vi "Mock Command.vi"(8 "error in (no error)":errorcluster, 11 "VISA Resource in":refnum<visa-resource-name>) -> (0 "error out":errorcluster, 1 "Fake Output":dbl, 3 "VISA Resource out":refnum<visa-resource-name>)   [LabVIEW 2020, in "plugin_flodx_pressure.lvlib" / "mock_driver.lvlib"]
doc: "Example of a mock or dummy driver VI which is meant to be called within plugin.lvlib in place of real instrument drivers as a development/debugging tool where hardware access may not be possible or convienent."
uses:
  mock_driver.lvlib
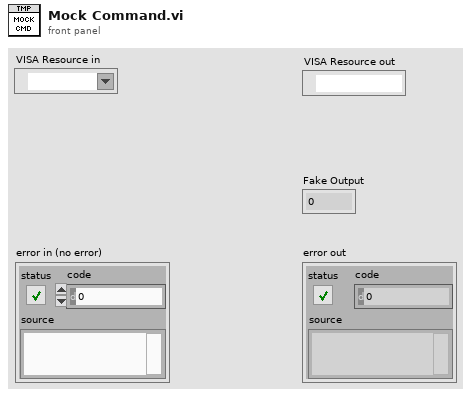
[diagram p1: front panel]
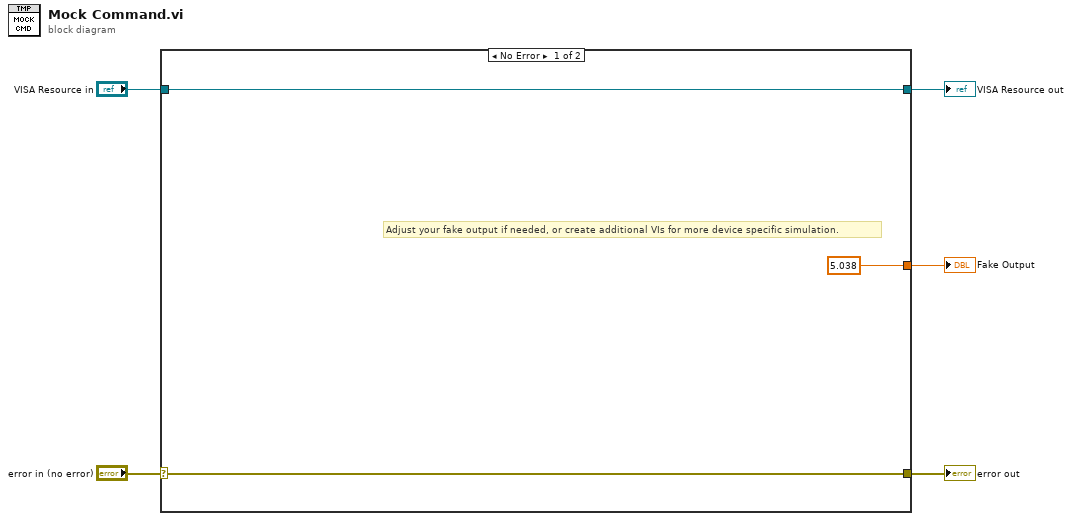
[diagram p0: block diagram]
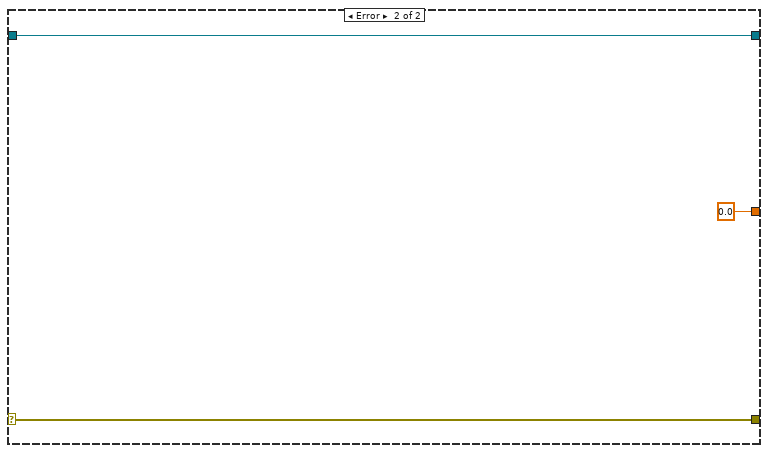
[diagram p2: hidden frame]
diagram:
  n1 = case shown="No Error" "error in (no error)" {
    selector: "error in (no error)" -> [w7 w10]
    tunnel: "VISA Resource in" -> [w8 w11]
    tunnel: [w8 w11] -> w4
    tunnel: [w7 w10] -> w2
    tunnel: [5.038 ("pH") 0.0 ("pH")] -> w1
    frame No Error {
      # "Adjust your fake output if needed, or create additional VIs for more device specific simulation."
    }
    frame Error {
    }
  }
  "VISA Resource out" <- w4
  "error out" <- w2
  "Fake Output" <- w1
